vi "trafficlightv3_state_machine.vi"() -> ()   [LabVIEW 2025]
uses:
  <vilib>/MakerHub/LINX/Public/Peripherals/Digital/Digital Write 1 Chan.vi
  <vilib>/MakerHub/LINX/Public/Peripherals/Digital/Digital Write N Chans.vi
  <vilib>/MakerHub/LINX/Private/Local IO/LinxDigitalWrite.vi
  <vilib>/MakerHub/LINX/Public/Utilities/Check Channel.vi
  <vilib>/MakerHub/LINX/Public/Utilities/Open Serial.vi
  <vilib>/httpClient/POSTBuffer.vi
  <vilib>/MakerHub/LINX/Private/Utilties/Generate Error.vi
  <vilib>/httpClient/LabVIEWHTTPClient.lvlib
  <vilib>/MakerHub/LINX/LMH-LINX.lvlib
panel:
  out "body":string
  out "match substring":string
  in  "stop":bool
  in  "D G":bool
  in  "D Y":bool
  in  "D R":bool
  in  "C G":bool
  in  "C Y":bool
  in  "C R":bool
  in  "B G":bool
  in  "B Y":bool
  in  "B R":bool
  in  "A G":bool
  in  "A Y":bool
  in  "A R":bool
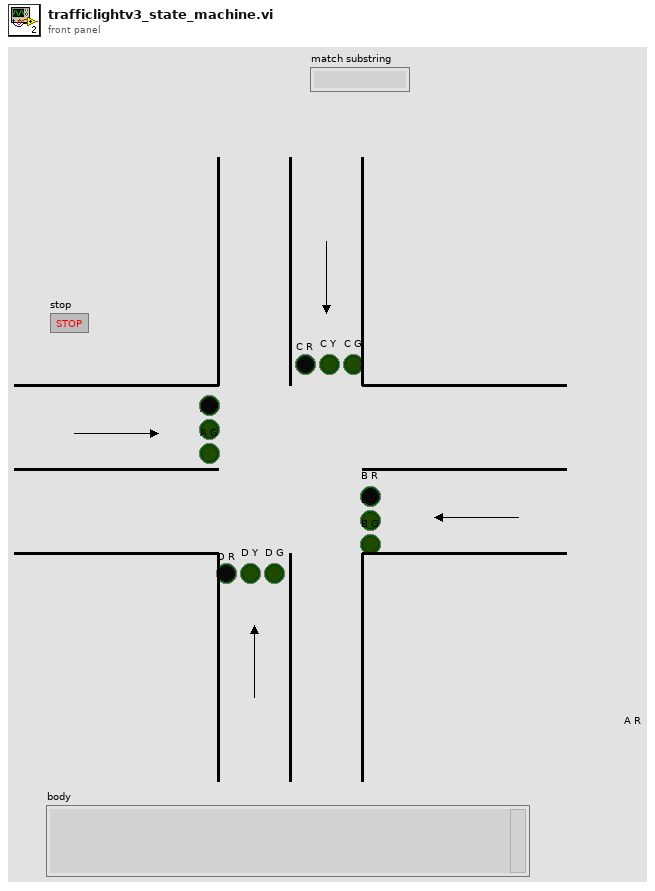
[diagram p1: front panel]
types:
  T1 = enum16{"H_YELLOW", "H_GREEN", "V_YELLOW", "V_GREEN", "CHECK _SIREN", "SIREN", ""}
  T2 = typedef "LMH-LINX.lvlib/LINX Ref.ctl" = cluster{"IO":T3, "Interface":T4, "LINX Device Config":T5}
  T3 = typedef "LMH-LINX.lvlib/Platform.ctl" = enum16{"Remote", "Local"}
  T4 = typedef "LMH-LINX.lvlib/Interface.ctl" = enum16{"Serial", "TCP"}
  T5 = typedef "LMH-LINX.lvlib/Device.lvlib/LINX Device Config.ctl" = cluster{"Interface":T4, "COM Port":refnum<visa-resource-name>, "TCP Configuration":T6, "Device Family":u8, "Device ID":u8, "Device Name":string, "TCP Ref":refnum<k5>, "Channels":T7}
  T6 = typedef "LMH-LINX.lvlib/Device.lvlib/TCP Config.ctl" = cluster{"IP Address":string, "Port":u16}
  T7 = typedef "LMH-LINX.lvlib/Channels.ctl" = cluster{"DI":u8[], "DO":u8[], "AI":u8[], "AO":u8[], "PWM":u8[], "QE":u8[], "UART":u8[], "I2C 2":u8[], "SPI":u8[], "CAN":u8[], "Servo":u8[], "AI Ref (V)":dbl, "AI Resolution (Bits)":u8, "AO Ref (V)":dbl, "AO Resolution (Bits)":u8}
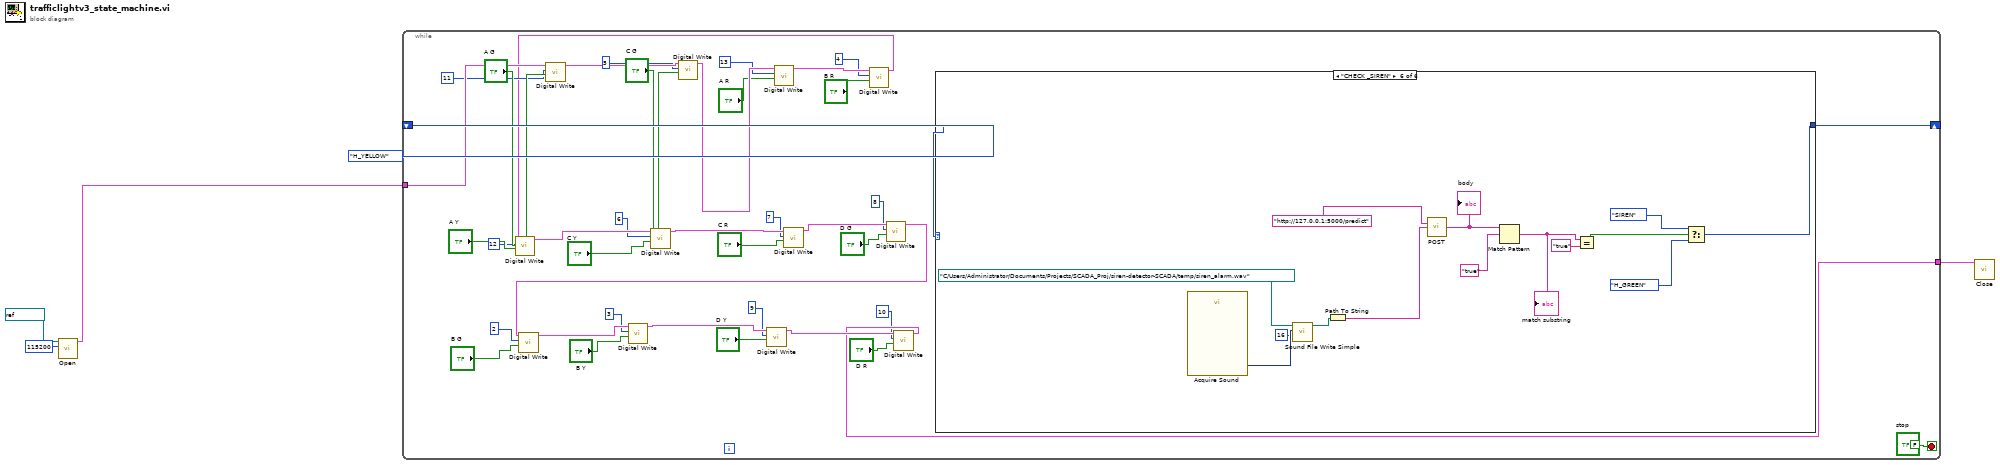
[diagram p0: block diagram]
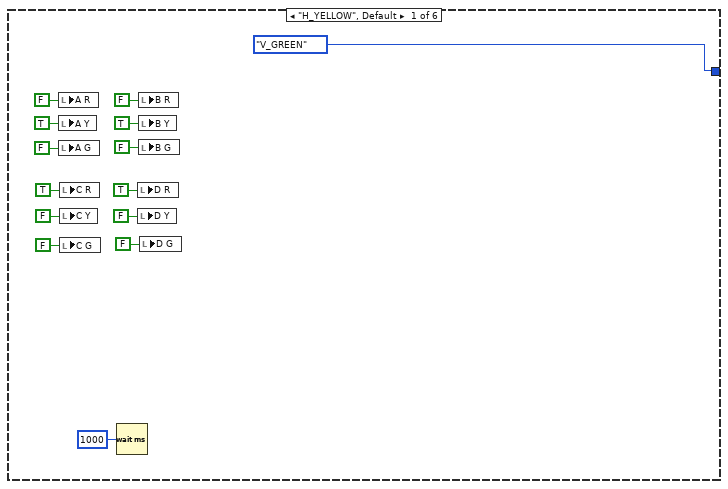
[diagram p2: hidden frame]
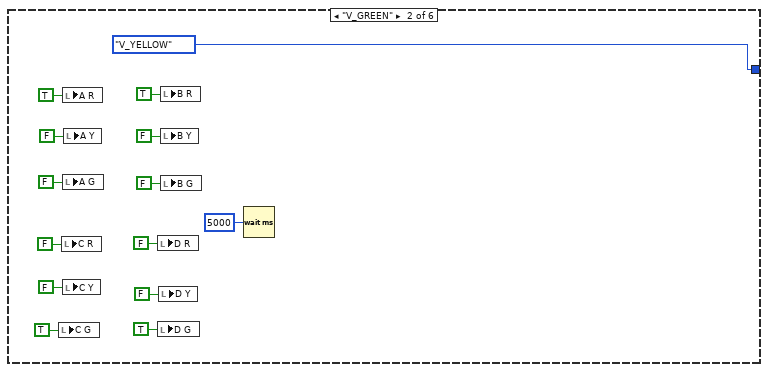
[diagram p3: hidden frame]
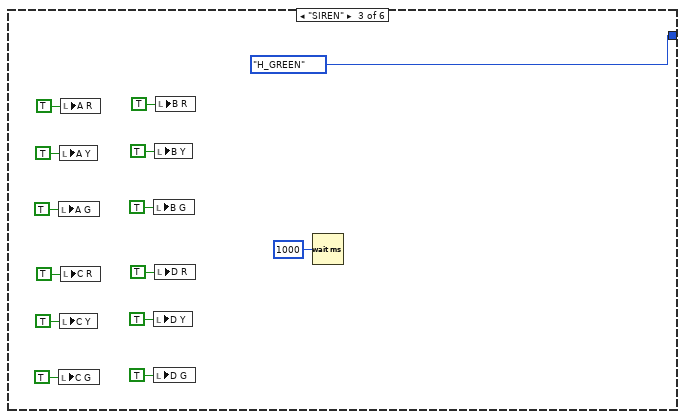
[diagram p4: hidden frame]
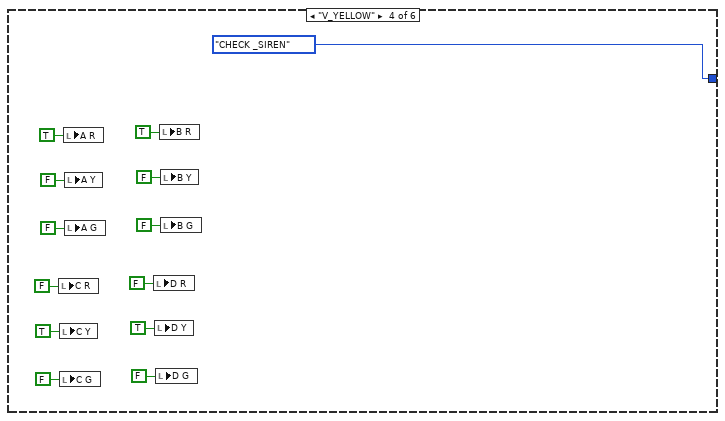
[diagram p5: hidden frame]
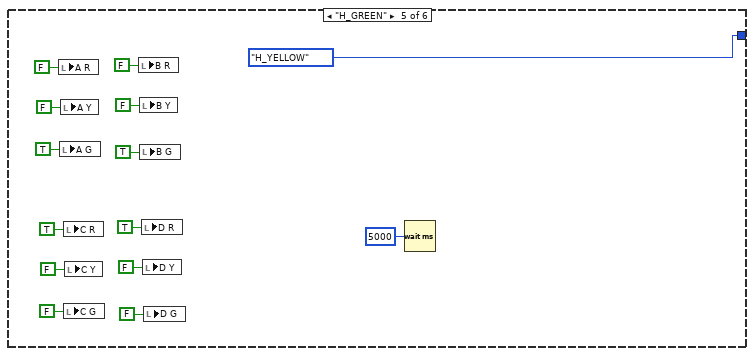
[diagram p6: hidden frame]
diagram:
  n1 = call-poly <vilib>:"Open.vi"("Baud Rate Override"=u32 115200, "Serial Port"=refnum<visa-resource-name> "COM5") -> ("LINX Resource"=w2:T2)  [unwired: 7 in, 2 out]
  n2 = while {
    shift-right: [w43] -> _
    shift-left: T1."H_YELLOW" -> [w44]
    tunnel: w2 -> [w42]
    tunnel: [w22] -> w1
    stop <- FALSE stop-if-true
    n3 = call-poly <vilib>:"Digital Write.vi"("Output Value"="A G", "DO Channel"=u8 11, "LINX Resource"=w42) -> ("LINX Resource"=w41:T2)  [unwired: 7 in, 1 out]
    n4 = call-poly <vilib>:"Digital Write.vi"("Output Value"="C G", "DO Channel"=u8 5, "LINX Resource"=w41) -> ("LINX Resource"=w36:T2)  [unwired: 7 in, 1 out]
    n5 = call-poly <vilib>:"Digital Write.vi"("Output Value"="A R", "DO Channel"=u8 13, "LINX Resource"=w36) -> ("LINX Resource"=w35:T2)  [unwired: 7 in, 1 out]
    n6 = call-poly <vilib>:"Digital Write.vi"("Output Value"="B R", "DO Channel"=u8 4, "LINX Resource"=w35) -> ("LINX Resource"=w30:T2)  [unwired: 7 in, 1 out]
    n7 = call-poly <vilib>:"Digital Write.vi"("Output Value"="A Y", "DO Channel"=u8 12, "LINX Resource"=w30) -> ("LINX Resource"=w29:T2)  [unwired: 7 in, 1 out]
    n8 = call-poly <vilib>:"Digital Write.vi"("Output Value"="C Y", "DO Channel"=u8 6, "LINX Resource"=w29) -> ("LINX Resource"=w28:T2)  [unwired: 7 in, 1 out]
    n9 = call-poly <vilib>:"Digital Write.vi"("Output Value"="C R", "DO Channel"=u8 7, "LINX Resource"=w28) -> ("LINX Resource"=w27:T2)  [unwired: 7 in, 1 out]
    n10 = call-poly <vilib>:"Digital Write.vi"("Output Value"="D G", "DO Channel"=u8 8, "LINX Resource"=w27) -> ("LINX Resource"=w26:T2)  [unwired: 7 in, 1 out]
    n11 = call-poly <vilib>:"Digital Write.vi"("Output Value"="B G", "DO Channel"=u8 2, "LINX Resource"=w26) -> ("LINX Resource"=w25:T2)  [unwired: 7 in, 1 out]
    n12 = call-poly <vilib>:"Digital Write.vi"("Output Value"="B Y", "DO Channel"=u8 3, "LINX Resource"=w25) -> ("LINX Resource"=w24:T2)  [unwired: 7 in, 1 out]
    n13 = call-poly <vilib>:"Digital Write.vi"("Output Value"="D Y", "DO Channel"=u8 9, "LINX Resource"=w24) -> ("LINX Resource"=w23:T2)  [unwired: 7 in, 1 out]
    n14 = call-poly <vilib>:"Digital Write.vi"("Output Value"="D R", "DO Channel"=u8 10, "LINX Resource"=w23) -> ("LINX Resource"=w22:T2)  [unwired: 7 in, 1 out]
    n15 = case shown="\"CHECK _SIREN\"" w44 {
      tunnel: [T1."V_GREEN" T1."V_YELLOW" T1."H_GREEN" T1."CHECK _SIREN" T1."H_YELLOW" w126] -> w43
      frame "H_YELLOW", Default {
        n16 = local write "A R"(FALSE ("A R")) -> ()
        n17 = local write "A Y"(TRUE ("A Y")) -> ()
        n18 = local write "A G"(FALSE ("A G")) -> ()
        n19 = local write "C R"(TRUE ("C R")) -> ()
        n20 = local write "C Y"(FALSE ("C Y")) -> ()
        n21 = local write "C G"(FALSE ("C G")) -> ()
        n22 = Wait (ms)(milliseconds to wait=u32 1000) -> ()  [unwired: 1 out]
        n23 = local write "D R"(TRUE ("D R")) -> ()
        n24 = local write "D Y"(FALSE ("D Y")) -> ()
        n25 = local write "B R"(FALSE ("B R")) -> ()
        n26 = local write "B Y"(TRUE ("B Y")) -> ()
        n27 = local write "B G"(FALSE ("B G")) -> ()
        n28 = local write "D G"(FALSE ("D G")) -> ()
      }
      frame "V_GREEN" {
        n29 = local write "C G"(TRUE ("C G")) -> ()
        n30 = local write "C R"(FALSE ("C R")) -> ()
        n31 = local write "A R"(TRUE ("A R")) -> ()
        n32 = local write "A G"(FALSE ("A G")) -> ()
        n33 = local write "C Y"(FALSE ("C Y")) -> ()
        n34 = local write "A Y"(FALSE ("A Y")) -> ()
        n35 = local write "D R"(FALSE ("D R")) -> ()
        n36 = local write "D G"(TRUE ("D G")) -> ()
        n37 = local write "D Y"(FALSE ("D Y")) -> ()
        n38 = local write "B R"(TRUE ("B R")) -> ()
        n39 = local write "B Y"(FALSE ("B Y")) -> ()
        n40 = local write "B G"(FALSE ("B G")) -> ()
        n41 = Wait (ms)(milliseconds to wait=u32 5000) -> ()  [unwired: 1 out]
      }
      frame "SIREN" {
        n42 = local write "A G"(TRUE ("A G")) -> ()
        n43 = local write "C G"(TRUE ("C G")) -> ()
        n44 = local write "A Y"(TRUE ("A Y")) -> ()
        n45 = local write "C Y"(TRUE ("C Y")) -> ()
        n46 = local write "A R"(TRUE ("A R")) -> ()
        n47 = local write "C R"(TRUE ("C R")) -> ()
        n48 = local write "B G"(TRUE ("B G")) -> ()
        n49 = local write "D Y"(TRUE ("D Y")) -> ()
        n50 = local write "D G"(TRUE ("D G")) -> ()
        n51 = local write "B Y"(TRUE ("B Y")) -> ()
        n52 = local write "D R"(TRUE ("D R")) -> ()
        n53 = local write "B R"(TRUE ("B R")) -> ()
        n54 = Wait (ms)(milliseconds to wait=u32 1000) -> ()  [unwired: 1 out]
      }
      frame "V_YELLOW" {
        n55 = local write "C R"(FALSE ("C R")) -> ()
        n56 = local write "C Y"(TRUE ("C Y")) -> ()
        n57 = local write "C G"(FALSE ("C G")) -> ()
        n58 = local write "A R"(TRUE ("A R")) -> ()
        n59 = local write "A Y"(FALSE ("A Y")) -> ()
        n60 = local write "A G"(FALSE ("A G")) -> ()
        n61 = local write "D R"(FALSE ("D R")) -> ()
        n62 = local write "D Y"(TRUE ("D Y")) -> ()
        n63 = local write "D G"(FALSE ("D G")) -> ()
        n64 = local write "B R"(TRUE ("B R")) -> ()
        n65 = local write "B Y"(FALSE ("B Y")) -> ()
        n66 = local write "B G"(FALSE ("B G")) -> ()
      }
      frame "H_GREEN" {
        n67 = local write "A R"(FALSE ("A R")) -> ()
        n68 = local write "A G"(TRUE ("A G")) -> ()
        n69 = local write "A Y"(FALSE ("A Y")) -> ()
        n70 = local write "C R"(TRUE ("C R")) -> ()
        n71 = local write "C G"(FALSE ("C G")) -> ()
        n72 = local write "C Y"(FALSE ("C Y")) -> ()
        n73 = local write "B R"(FALSE ("B R")) -> ()
        n74 = local write "B Y"(FALSE ("B Y")) -> ()
        n75 = local write "B G"(TRUE ("B G")) -> ()
        n76 = local write "D R"(TRUE ("D R")) -> ()
        n77 = local write "D Y"(FALSE ("D Y")) -> ()
        n78 = local write "D G"(FALSE ("D G")) -> ()
        n79 = Wait (ms)(milliseconds to wait=u32 5000) -> ()  [unwired: 1 out]
      }
      frame "CHECK _SIREN" {
        n80 = call "Acquire Sound"() -> ("Data"=w125:dynamicdata)  [unwired: 18 in, 1 out]
        n81 = call <vilib>:"Sound File Write Simple.vi"("bits per sample"=16, "data"=w125, "path"=path "C:/Users/Administrator/Documents/Projects/SCADA_Proj/siren-detector-SCADA/temp/siren_alarm.wav") -> ("path out"=w117:path)  [unwired: 7 in, 1 out]
        n82 = Path To String(path=w117) -> (string=w116:string)
        n83 = call-poly <vilib>:"POST.vi"("url"="http://127.0.0.1:5000/predict", "buffer"=w116) -> ("body"=w115:string)  [unwired: 10 in, 3 out]
        "body" <- w115
        n84 = Match Pattern(string=w115, regular expression="true") -> (match substring=w120:string)  [unwired: 1 in, 3 out]
        "match substring" <- w120
        n85 = Equal?(x=w120, y="true") -> (x = y?=w118:bool)
        n86 = Select(t=T1."SIREN", s=w118, f=T1."H_GREEN") -> (s? t:f=w126:T1)
      }
    }
  }
  n87 = call <vilib>:"Close.vi"("LINX Resource"=w1) -> ()  [unwired: 10 in, 1 out]
